vi "PAM.vi"() -> ()   [LabVIEW 2013]
uses:
  <vilib>/express/express analysis/Spectral/Block/exnSpectralBlock spectral measurements RMS poly.vi
  <vilib>/express/express analysis/Spectral/Block/exnSpectralBlock spectral measurements RMS DDT.vi
  <vilib>/express/express analysis/Spectral/XNode/ExpressSpectralMeasurementsBlockNode.xnode
panel:
  out "Waveform Graph 3":dynamicdata(graph)
  out "Waveform Graph 2":dynamicdata(graph)
  out "Waveform Graph":dynamicdata(graph)
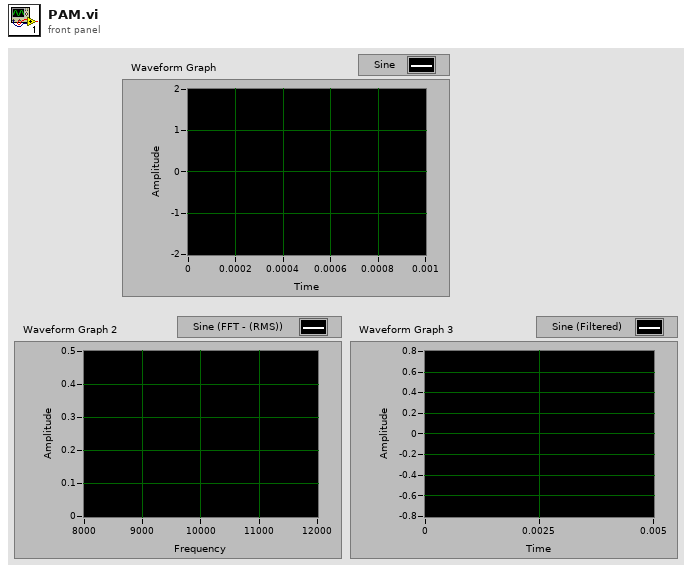
[diagram p1: front panel]
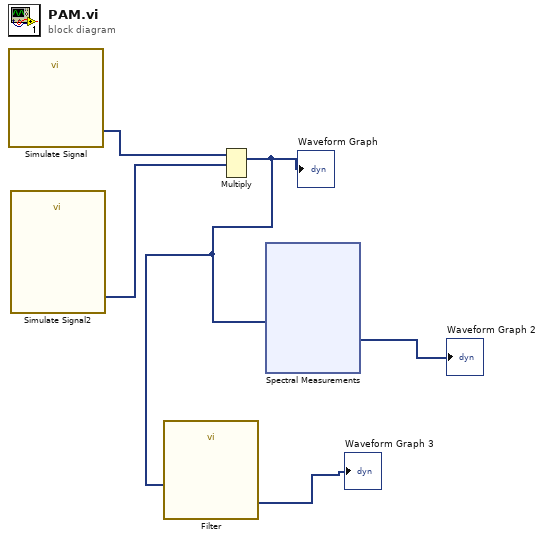
[diagram p0: block diagram]
diagram:
  n1 = call "Simulate Signal"() -> ("Sine"=w5:dynamicdata)  [unwired: 14 in, 1 out]
  n2 = call "Simulate Signal2"() -> ("Square"=w4:dynamicdata)  [unwired: 14 in, 1 out]
  n3 = Multiply(1:w4, 2:w5) -> (0:w2:dynamicdata)  [unwired: 1 in, 1 out]
  "Waveform Graph" <- w2
  n4 = call "Filter"("Signal"=w2) -> ("Filtered Signal"=→"Waveform Graph 3":dynamicdata)  [unwired: 9 in, 1 out]
  n5 = xnode "Spectral Measurements"("Signals"=w2) -> ("FFT - (RMS)"=→"Waveform Graph 2":dynamicdata)  [unwired: 1 in, 2 out]
